vi "Samle qsns practice 20.vi"() -> ()   [LabVIEW 2020]
panel:
  out "appended array":dbl[][](array[numeric])
  out "subarray":dbl[](array[numeric])
  out "Numeric":i32
  out "x*y":dbl
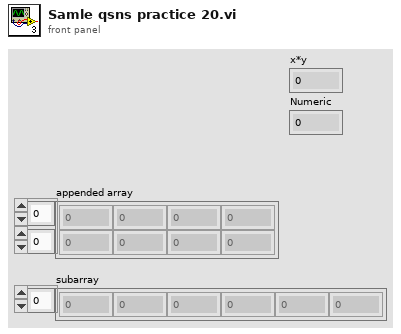
[diagram p1: front panel]
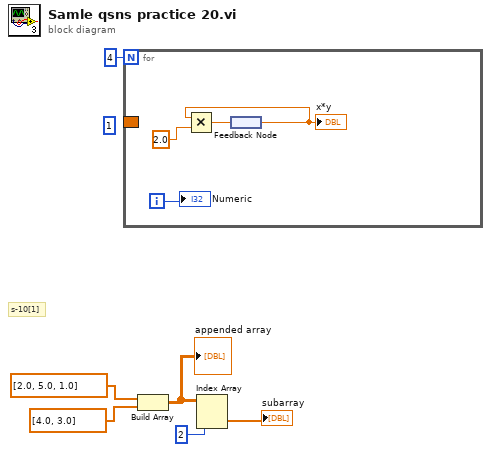
[diagram p0: block diagram]
diagram:
  (unwired) 1
  # "s-10[1]"
  n1 = for {
    N: 4 -> [_]
    border: _ -> [_]
    i -> [w9]
    n2 = feedback #1() -> (w7:dbl)
    "x*y" <- w7
    n3 = Multiply(x=w7, y=2.0) -> (x*y=w8:dbl)
    n4 = feedback-in #1(w8) -> ()
    "Numeric" <- w9
  }
  n5 = Build Array(dbl[] [2.0, 5.0, 1.0], dbl[] [4.0, 3.0]) -> (w3:dbl[][])
  "appended array" <- w3
  n6 = Index Array(array=w3, index (col)=2 ("disabled index (col)")) -> (element=→"subarray":dbl[])  [unwired: 1 in]
